vi "Get All Available.vi"(8 "error in":errorcluster, 10 "all rows":string[][](array[string])) -> (0 "error out":errorcluster, 3 "Available Parameters":T1)   [LabVIEW 2013]
doc: "This VI inputs all data from the comm map file and outputs a cluster of arrays containing the available parameters for each protocol."
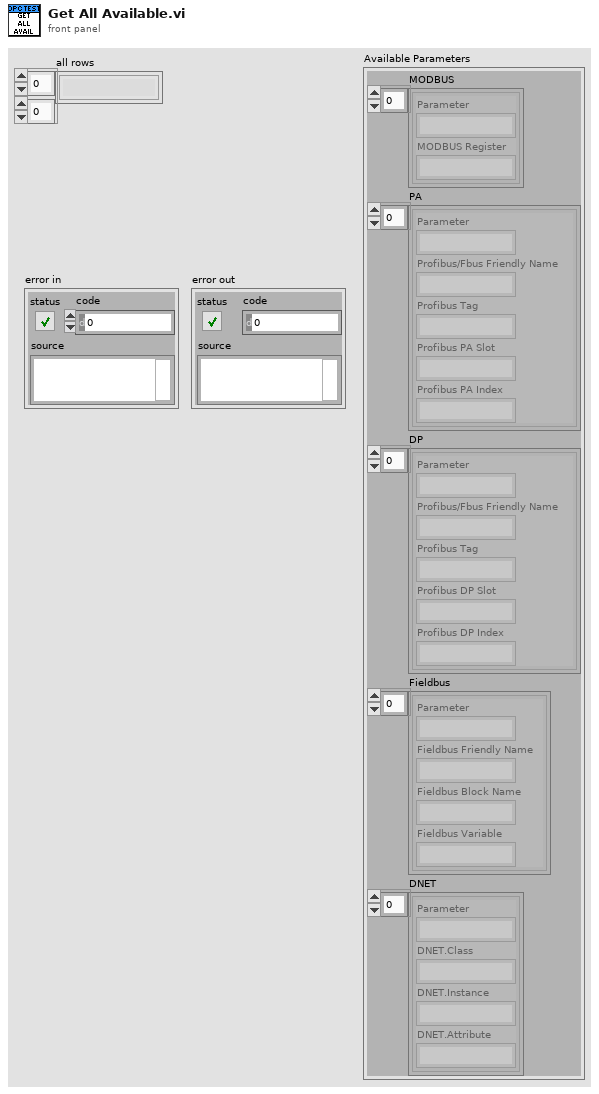
[diagram p1: front panel]
types:
  T1 = cluster{"MODBUS":cluster{"Parameter":string, "MODBUS Register":string}[], "PA":cluster{"Parameter":string, "Profibus/Fbus Friendly Name":string, "Profibus Tag":string, "Profibus PA Slot":string, "Profibus PA Index":string}[], "DP":cluster{"Parameter":string, "Profibus/Fbus Friendly Name":string, "Profibus Tag":string, "Profibus DP Slot":string, "Profibus DP Index":string}[], "Fieldbus":cluster{"Parameter":string, "Fieldbus Friendly Name":string, "Fieldbus Block Name":string, "Fieldbus Variable":string}[], "DNET":cluster{"Parameter":string, "DNET.Class":string, "DNET.Instance":string, "DNET.Attribute":string}[]}
  T2 = cluster{"Parameter":string, "DNET.Class":string, "DNET.Instance":string, "DNET.Attribute":string}
  T3 = cluster{"Parameter":string, "Fieldbus Friendly Name":string, "Fieldbus Block Name":string, "Fieldbus Variable":string}
  T4 = cluster{"Parameter":string, "Profibus/Fbus Friendly Name":string, "Profibus Tag":string, "Profibus DP Slot":string, "Profibus DP Index":string}
  T5 = cluster{"Parameter":string, "Profibus/Fbus Friendly Name":string, "Profibus Tag":string, "Profibus PA Slot":string, "Profibus PA Index":string}
  T6 = cluster{"Parameter":string, "MODBUS Register":string}
  T7 = cluster{"Parameter":string, "MODBUS Register":string}[]
  T8 = cluster{"Parameter":string, "Profibus/Fbus Friendly Name":string, "Profibus Tag":string, "Profibus PA Slot":string, "Profibus PA Index":string}[]
  T9 = cluster{"Parameter":string, "Profibus/Fbus Friendly Name":string, "Profibus Tag":string, "Profibus DP Slot":string, "Profibus DP Index":string}[]
  T10 = cluster{"Parameter":string, "Fieldbus Friendly Name":string, "Fieldbus Block Name":string, "Fieldbus Variable":string}[]
  T11 = cluster{"Parameter":string, "DNET.Class":string, "DNET.Instance":string, "DNET.Attribute":string}[]
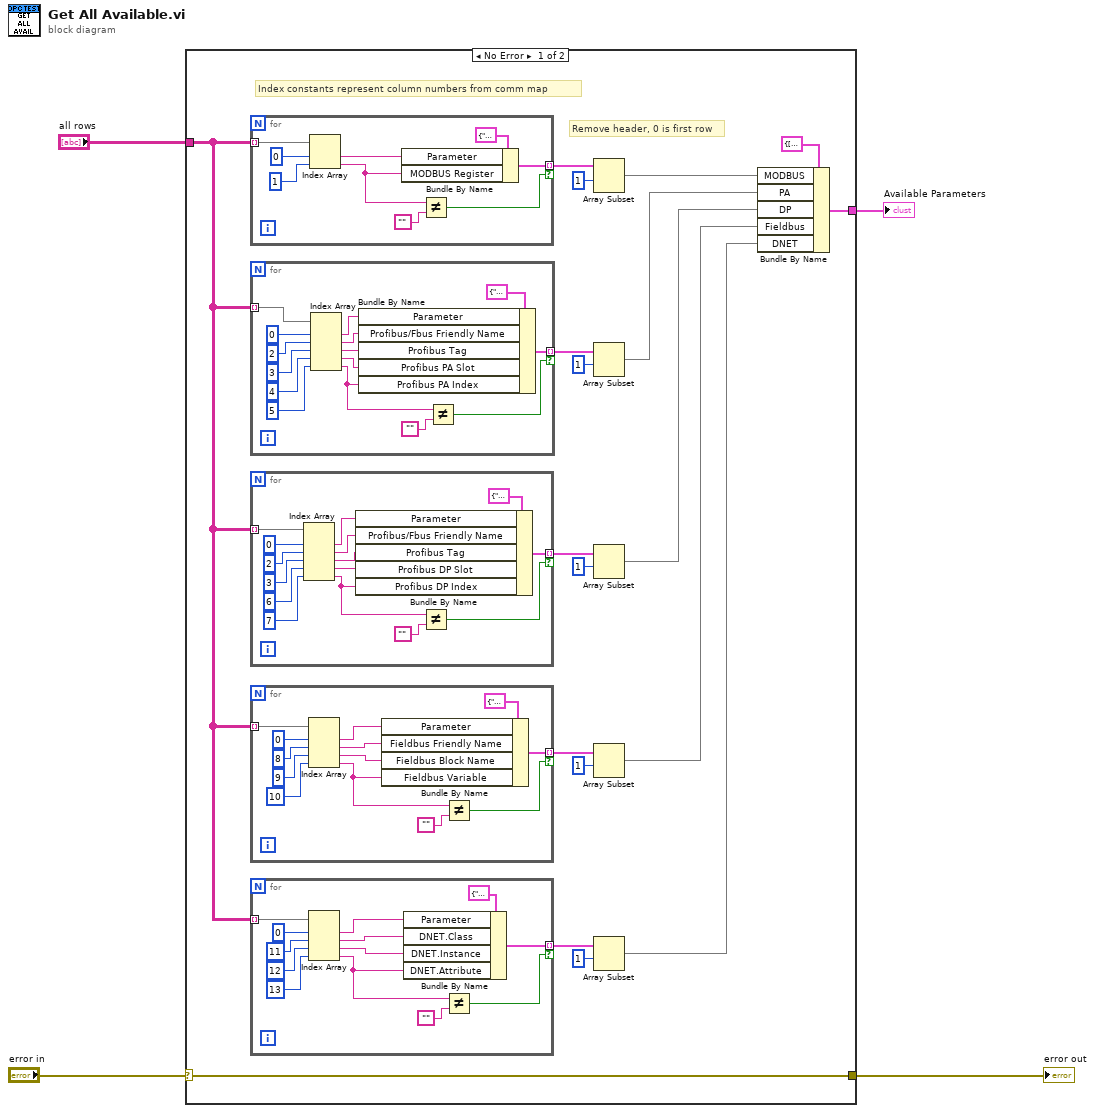
[diagram p0: block diagram]
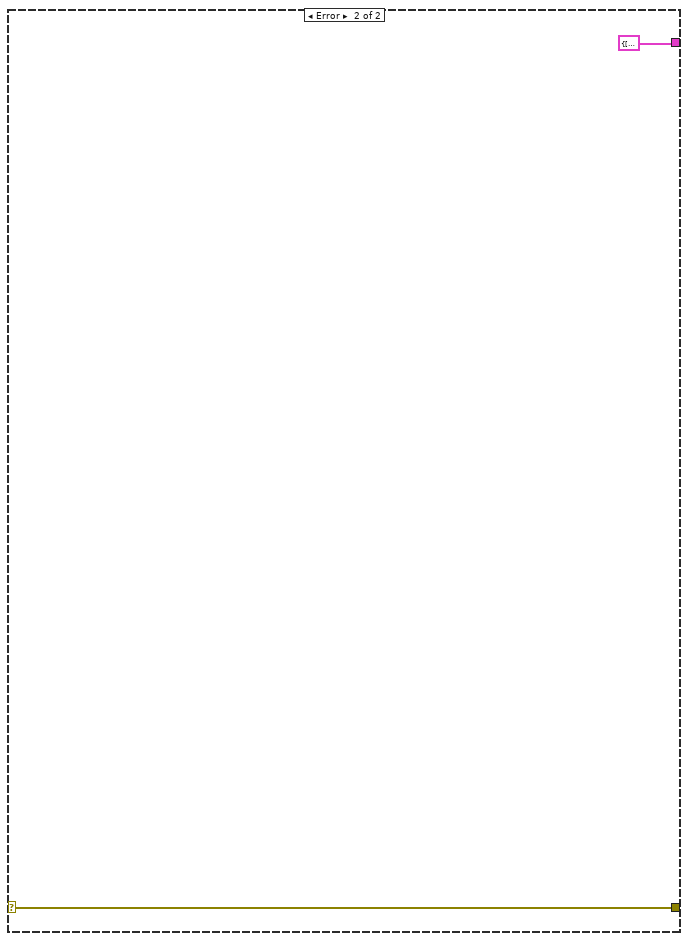
[diagram p2: hidden frame]
diagram:
  n1 = case shown="No Error" "error in" {
    selector: "error in" -> [w9 w90]
    tunnel: [w9 w90] -> w3
    tunnel: "all rows" -> [w6 _]
    tunnel: [w5 T1 {"MODBUS"=[], "PA"=[], "DP"=[], "Fieldbus"=[], "DNET"=[]} ("Available Parameters")] -> w1
    frame No Error {
      # "Index constants represent column numbers from comm map"
      # "Remove header, 0 is first row"
      n2 = for {
        tunnel: w6 -> [w88] mode=indexing
        tunnel: [w85] -> w10 mode=indexing if=w82
        n3 = Index Array(array=w88, index #1=0 ("index"), index #2=1 ("index")) -> (element #1=w86:string, element #2=w84:string)
        n4 = Bundle By Name(cluster=T6 {"Parameter"="", "MODBUS Register"=""} ("MODBUS"), "Parameter"=w86, "MODBUS Register"=w84) -> (w85:T6)
        n5 = Not Equal?(x=w84, y="") -> (x != y?=w82:bool)
      }
      n6 = for {
        tunnel: w6 -> [w79] mode=indexing
        tunnel: [w77] -> w11 mode=indexing if=w74
        n7 = Index Array(array=w79, index #1=0 ("index"), index #2=2 ("index"), index #3=3 ("index"), index #4=4 ("index"), index #5=5 ("index")) -> (element #1=w78:string, element #2=w76:string, element #3=w71:string, element #4=w70:string, element #5=w65:string)
        n8 = Bundle By Name(cluster=T5 {"Parameter"="", "Profibus/Fbus Friendly Name"="", "Profibus Tag"="", "Profibus PA Slot"="", "Profibus PA Index"=""} ("Profibus PA"), "Parameter"=w78, "Profibus/Fbus Friendly Name"=w76, "Profibus Tag"=w71, "Profibus PA Slot"=w70, "Profibus PA Index"=w65) -> (w77:T5)
        n9 = Not Equal?(x=w65, y="") -> (x != y?=w74:bool)
      }
      n10 = for {
        tunnel: w6 -> [w64] mode=indexing
        tunnel: [w63] -> w12 mode=indexing if=w61
        n11 = Index Array(array=w64, index #1=0 ("index"), index #2=2 ("index"), index #3=3 ("index"), index #4=6 ("index"), index #5=7 ("index")) -> (element #1=w59:string, element #2=w58:string, element #3=w57:string, element #4=w56:string, element #5=w55:string)
        n12 = Bundle By Name(cluster=T4 {"Parameter"="", "Profibus/Fbus Friendly Name"="", "Profibus Tag"="", "Profibus DP Slot"="", "Profibus DP Index"=""} ("Profibus PA"), "Parameter"=w59, "Profibus/Fbus Friendly Name"=w58, "Profibus Tag"=w57, "Profibus DP Slot"=w56, "Profibus DP Index"=w55) -> (w63:T4)
        n13 = Not Equal?(x=w55, y="") -> (x != y?=w61:bool)
      }
      n14 = for {
        tunnel: w6 -> [w49] mode=indexing
        tunnel: [w47] -> w19 mode=indexing if=w44
        n15 = Index Array(array=w49, index #1=0 ("index"), index #2=8 ("index"), index #3=9 ("index"), index #4=10 ("index")) -> (element #1=w48:string, element #2=w46:string, element #3=w42:string, element #4=w41:string)
        n16 = Bundle By Name(cluster=T3 {"Parameter"="", "Fieldbus Friendly Name"="", "Fieldbus Block Name"="", "Fieldbus Variable"=""} ("Fildbus"), "Parameter"=w48, "Fieldbus Friendly Name"=w46, "Fieldbus Block Name"=w42, "Fieldbus Variable"=w41) -> (w47:T3)
        n17 = Not Equal?(x=w41, y="") -> (x != y?=w44:bool)
      }
      n18 = for {
        tunnel: w6 -> [w36] mode=indexing
        tunnel: [w34] -> w18 mode=indexing if=w31
        n19 = Index Array(array=w36, index #1=0 ("index"), index #2=11 ("index"), index #3=12 ("index"), index #4=13 ("index")) -> (element #1=w35:string, element #2=w33:string, element #3=w30:string, element #4=w29:string)
        n20 = Bundle By Name(cluster=T2 {"Parameter"="", "DNET.Class"="", "DNET.Instance"="", "DNET.Attribute"=""} ("DNET"), "Parameter"=w35, "DNET.Class"=w33, "DNET.Instance"=w30, "DNET.Attribute"=w29) -> (w34:T2)
        n21 = Not Equal?(x=w29, y="") -> (x != y?=w31:bool)
      }
      n22 = Array Subset(array=w10, index=1) -> (w20:T7)  [unwired: 1 in]
      n23 = Array Subset(array=w11, index=1) -> (w21:T8)  [unwired: 1 in]
      n24 = Array Subset(array=w12, index=1) -> (w7:T9)  [unwired: 1 in]
      n25 = Array Subset(array=w19, index=1) -> (w22:T10)  [unwired: 1 in]
      n26 = Array Subset(array=w18, index=1) -> (w23:T11)  [unwired: 1 in]
      n27 = Bundle By Name(cluster=T1 {"MODBUS"=[], "PA"=[], "DP"=[], "Fieldbus"=[], "DNET"=[]} ("Available Parameters"), "MODBUS"=w20, "PA"=w21, "DP"=w7, "Fieldbus"=w22, "DNET"=w23) -> (w5:T1)
    }
    frame Error {
    }
  }
  "error out" <- w3
  "Available Parameters" <- w1
